vi "Send Single Trigger.vi"(8 "error in (no error)":errorcluster, 11 "VNA-ZNB in":refnum<class "VNA-ZNB.lvclass">) -> (0 "error out":errorcluster, 3 "VNA-ZNB out":refnum<class "VNA-ZNB.lvclass">)   [LabVIEW 2020, in "VNA-ZNB.lvclass"]
doc: "Sent a single trigger for the VNA. It uses the OPC command to wait until completion.\nIt will use (sweeptime * N average * N ports) for the VISA timeout."
uses:
  VNA-ZNB.lvclass
  C:/Sandbox/Git_Sandbox/WiSpry Test Framework source code (LV20)/WiSpry Test Framework/Instruments/Vector Network Analyzer/Vector Network Analyzer.lvclass
  C:/Sandbox/Git_Sandbox/WiSpry Test Framework source code (LV20)/WiSpry Test Framework/Instruments/Instrument.lvclass
  Instrument.lvclass/Instrument.ctl
  Vector Network Analyzer.lvclass/Vector Network Analyzer.ctl
  Vector Network Analyzer.lvclass
  Instrument.lvclass
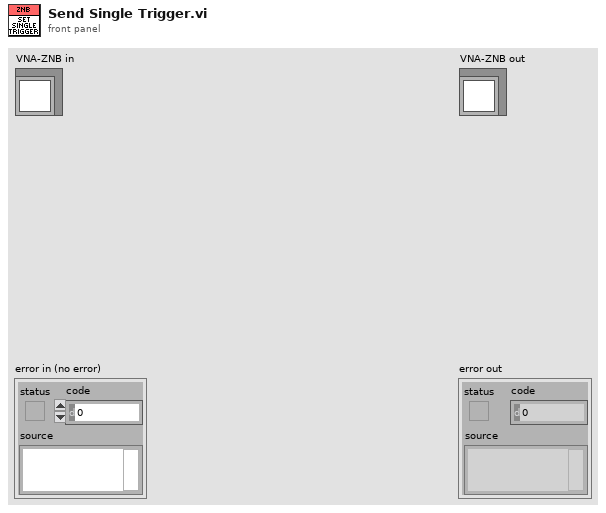
[diagram p1: front panel]
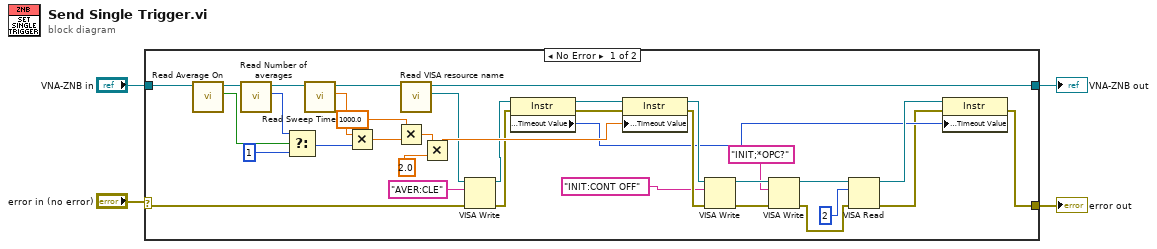
[diagram p0: block diagram]
diagram:
  n1 = case shown="No Error" "error in (no error)" {
    selector: "error in (no error)" -> [w5 w41]
    tunnel: "VNA-ZNB in" -> [w39 w40]
    tunnel: [w25 w40] -> w2
    tunnel: [w16 w41] -> w1
    frame No Error {
      n2 = call "Read Average On.vi"("Vector Network Analyzer in"=w39) -> ("Average On"=w35:bool, "Vector Network Analyzer out"=w38:refnum<class "VNA-ZNB.lvclass">)  [unwired: 9 in]
      n3 = call "Read Number of averages.vi"("Vector Network Analyzer in"=w38) -> ("Number of averages"=w36:i32, "Vector Network Analyzer out"=w37:refnum<class "VNA-ZNB.lvclass">)  [unwired: 9 in]
      n4 = Select(t=w36, s=w35, f=1) -> (s? t:f=w32:i32)
      n5 = call "Read Sweep Time.vi"("Vector Network Analyzer in"=w37) -> ("Sweep Time"=w33:dbl, "Vector Network Analyzer out"=w31:refnum<class "VNA-ZNB.lvclass">)  [unwired: 9 in]
      n6 = Multiply(x=w33, y=w32) -> (x*y=w28:dbl)
      n7 = Multiply(x=1000.0, y=w28) -> (x*y=w27:dbl)
      n8 = call "Read VISA resource name.vi"("Instrument in"=w31) -> ("VISA resource name"=w8:refnum<visa-resource-name>, "Instrument out"=w25:refnum<class "VNA-ZNB.lvclass">)  [unwired: 9 in]
      n9 = Multiply(x=w27, y=2.0) -> (x*y=w21:dbl)
      n10 = VISA Write(VISA resource name=w8, write buffer="AVER:CLE", error in (no error)=w5) -> (VISA resource name out=w7:refnum<visa-resource-name>, error out=w9:errorcluster)  [unwired: 1 out]
      n11 = property class="Instr"(reference=w7, error in=w9) -> (reference out=w30:refnum<visa-resource-name>, error out=w29:errorcluster, "General Settings:Timeout Value"=w18:u32)
      n12 = property class="Instr"(reference=w30, error in=w29, "General Settings:Timeout Value"=w21) -> (reference out=w24:refnum<visa-resource-name>, error out=w23:errorcluster)
      n13 = VISA Write(VISA resource name=w24, write buffer="INIT:CONT OFF", error in (no error)=w23) -> (VISA resource name out=w13:refnum<visa-resource-name>, error out=w14:errorcluster)  [unwired: 1 out]
      n14 = VISA Write(VISA resource name=w13, write buffer="INIT;*OPC?", error in (no error)=w14) -> (VISA resource name out=w12:refnum<visa-resource-name>, error out=w11:errorcluster)  [unwired: 1 out]
      n15 = VISA Read(VISA resource name=w12, byte count=u32 2, error in (no error)=w11) -> (VISA resource name out=w19:refnum<visa-resource-name>, error out=w17:errorcluster)  [unwired: 2 out]
      n16 = property class="Instr"(reference=w19, error in=w17, "General Settings:Timeout Value"=w18) -> (error out=w16:errorcluster)  [unwired: 1 out]
    }
    frame Error {
    }
  }
  "error out" <- w1
  "VNA-ZNB out" <- w2
